vi "Handle incomming messages.vi"(11 "module loopdata":T1) -> (0 "error out":errorcluster, 3 "OK":bool)   [LabVIEW 2019, in "Communication Interface.lvlib"]
uses:
  Communication Interface.lvlib
  module data.ctl
  Intertarget communication/CR_master_class/CR_master.lvclass
  Intertarget communication/CR slave_class/CR slave.lvclass
  SubVIs/Shared/CMD Read RX.ctl
  SubVIs/Shared/CMD Read RX index.ctl
  93a0a4a7-173a-43f5-bf28-7be2535433ae.vi
  48c2df5e-f12f-4e31-93d9-71ac4fdf9692.vi
  93a0a4a7-173a-43f5-bf28-7be2535433ae.vi/fab4b5b6-9762-4187-bffd-0adbcd2d5190.vi
  93a0a4a7-173a-43f5-bf28-7be2535433ae.vi/eb0db0a0-6387-48cc-9517-445619e830de.vi
  48c2df5e-f12f-4e31-93d9-71ac4fdf9692.vi/0a35ed28-1569-4b97-93b5-a089aa938873.vi
  48c2df5e-f12f-4e31-93d9-71ac4fdf9692.vi/d25f57df-6ce4-4576-a055-01dd08f6b6ca.vi
  <vilib>/Utility/High Resolution Relative Seconds.vi
  <vilib>/Utility/error.llb/Error Cluster From Error Code.vi
  SubVIs/Shared/System GV.vi
  <vilib>/addons/_JKI.lib/Serialization/JSON/Library/Unflatten From JSON String.vi
  <vilib>/ErrorRing/Error Ring.xnode
  SubVIs/IQBurst_memo_class/IQBurst_memo.lvclass
  Intertarget communication/CommandResponse communication.lvlib
  SubVIs/Shared/Shared.lvlib
  Data Managment/DataManagment.lvlib
  <vilib>/addons/_JKI.lib/Serialization/JSON/JKI JSON Serialization.lvlib
  Log/Log.lvlib
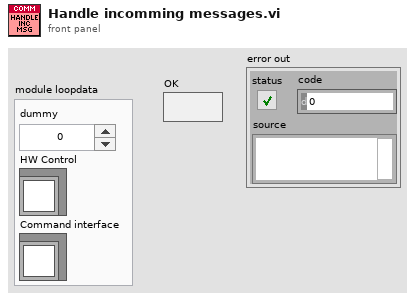
[diagram p1: front panel]
types:
  T1 = typedef "Communication Interface.lvlib/module data.ctl" = cluster{"dummy":dbl, "HW Control":refnum<class "CR_master.lvclass">, "Command interface":refnum<class "CR slave.lvclass">}
  T2 = typedef "Shared.lvlib/CMD Read RX.ctl" = cluster{"burst name":string}
  T3 = typedef "Shared.lvlib/CMD Read RX index.ctl" = cluster{"burst index":i32}
  T4 = typedef "Communication Interface.lvlib/message destination.ctl" = enum16{"unknown", "HW", "Data", "GUI", "Log", "Close"}
  T5 = cluster{"Boolean Round":bool, "code":i32, "source":string}
  T6 = typedef "DataManagment.lvlib/DM group info.ctl" = cluster{"group name":string, "burst names":string[], "burst sizes":dbl[], "Memory":dbl}
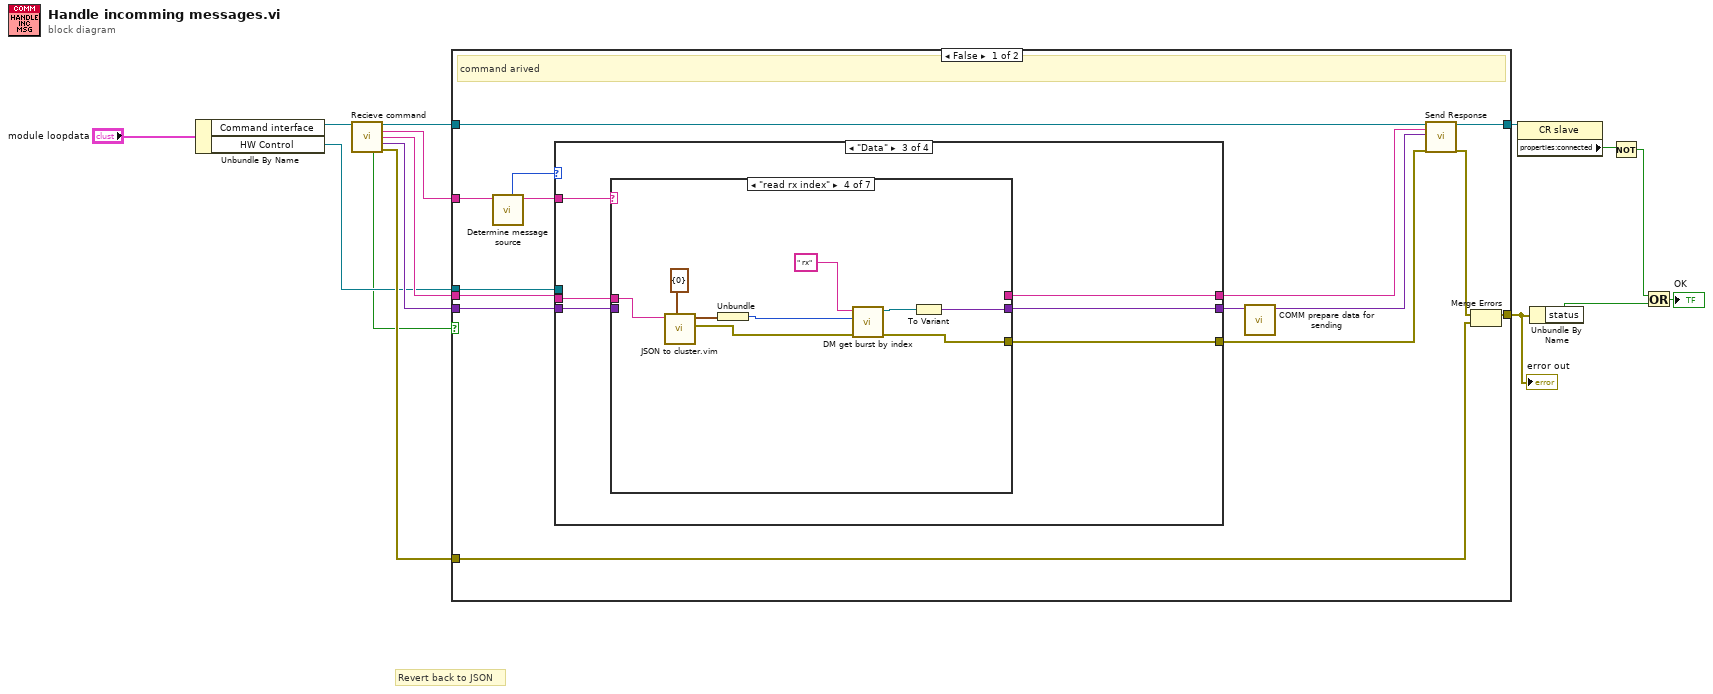
[diagram p0: block diagram]
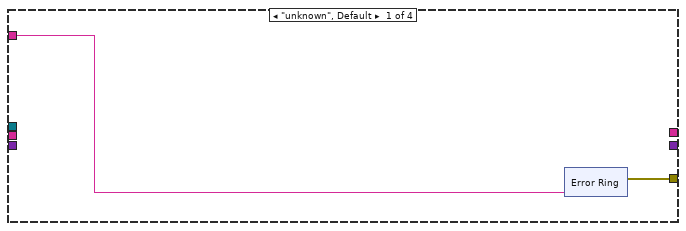
[diagram p2: hidden frame]
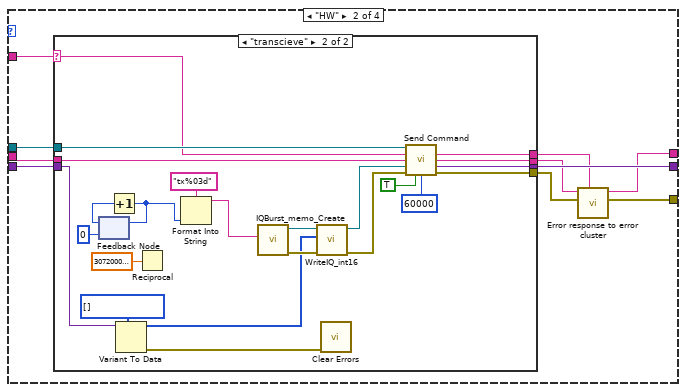
[diagram p3: hidden frame]
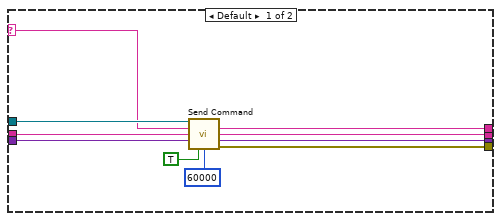
[diagram p4: hidden frame]
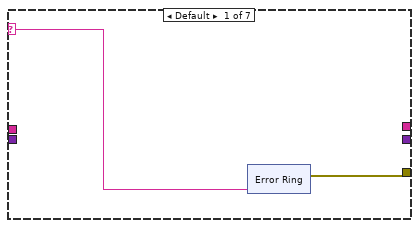
[diagram p5: hidden frame]
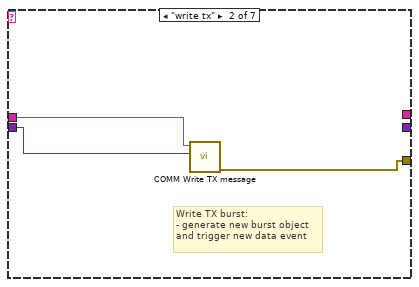
[diagram p6: hidden frame]
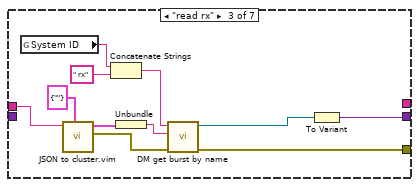
[diagram p7: hidden frame]
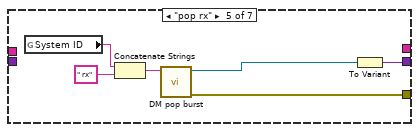
[diagram p8: hidden frame]
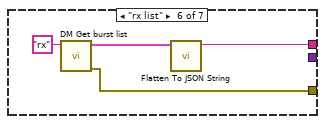
[diagram p9: hidden frame]
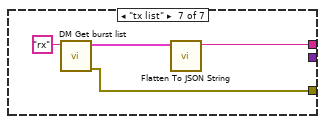
[diagram p10: hidden frame]
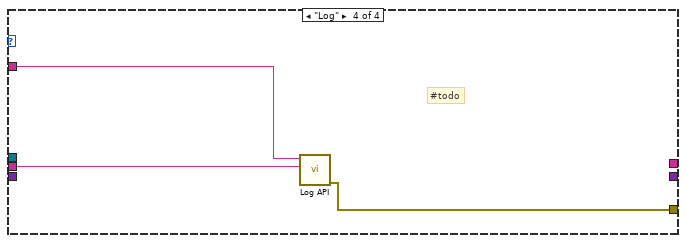
[diagram p11: hidden frame]
diagram:
  # "Revert back to JSON"
  n1 = Unbundle By Name("module loopdata") -> ("Command interface"=w2:refnum<class "CR slave.lvclass">, "HW Control"=w4:refnum<class "CR_master.lvclass">)
  n2 = call-dynamic "Recieve command.vi"("reference in"=w2) -> ("reference out"=w8:refnum<class "CR slave.lvclass">, "message"=w5:string, "parameters"=w6:string, "data"=w7:variant, "timed out?"=w3:bool, "error out"=w9:errorcluster)  [unwired: 9 in]
  n3 = case shown="False" w3 {
    tunnel: w4 -> [w30 _]
    tunnel: w5 -> [w23 _]
    tunnel: w6 -> [w29 _]
    tunnel: w7 -> [w28 _]
    tunnel: w8 -> [w27 w138]
    tunnel: w9 -> [w18 w139]
    tunnel: [w19 w139] -> w10
    tunnel: [w26 w138] -> w11
    frame False {
      # "command arived"
      n4 = call "Determine message source.vi"("message in"=w23) -> ("message out"=w22:string, "msg destination"=w21:T4)  [unwired: 9 in]
      n5 = case shown="\"Data\"" w21 {
        tunnel: w30 -> [_ w49 _ _]
        tunnel: w29 -> [_ w48 w86 w136]
        tunnel: w28 -> [_ w47 w87 _]
        tunnel: [_ w46 w84 _] -> w17
        tunnel: [_ w44 w83 _] -> w25
        tunnel: [w32 w43 w85 w135] -> w24
        tunnel: w22 -> [w31 w40 w88 w137]
        frame "unknown", Default {
          n6 = xnode "Error Ring"("parameter 0"=w31) -> ("error out"=w32:errorcluster)
        }
        frame "HW" {
          n7 = case shown="\"transcieve\"" w40 {
            selector: w40 -> [w50 w74]
            tunnel: w49 -> [w59 w82]
            tunnel: w48 -> [w58 w81]
            tunnel: w47 -> [w57 w66]
            tunnel: [w56 w80] -> w46
            tunnel: [w53 w77] -> w45
            tunnel: [w52 w76] -> w42
            tunnel: [w51 w75] -> w41
            frame Default {
              n8 = call-dynamic "Send Command.vi"("reference in"=w59, "message"=w50, "parameters"=w58, "data"=w57, "response?"=TRUE, "timeout"=60000) -> ("status"=w52:string, "reponse"=w53:string, "data"=w56:variant, "error out"=w51:errorcluster)  [unwired: 5 in, 1 out]
            }
            frame "transcieve" {
              n9 = feedback #1(0) -> (w65:i32)
              n10 = Increment(x=w65) -> (x+1=w63:i32)
              n11 = feedback-in #1(w63) -> ()
              n12 = Variant To Data(type=i16[] [], Variant=w66) -> (data=w61:i16[], error out=w73:errorcluster)  [unwired: 1 in]
              n13 = Reciprocal(x=3072000000.0 ("sample rate (Hz)")) -> ()  [unwired: 1 out]
              n14 = Format Into String(format string="tx%03d", w63) -> (resulting string=w72:string)  [unwired: 2 in, 1 out]
              n15 = call "IQBurst_memo_Create.vi"("burst name"=w72) -> ("error out"=w70:errorcluster, "reference out"=w71:refnum<class "IQBurst_memo.lvclass">)  [unwired: 9 in]
              n16 = call-dynamic "WriteIQ_int16.vi"("error in (no error)"=w70, "data"=w61, "reference in"=w71) -> ("error out"=w60:errorcluster, "reference out"=w62:refnum<class "IQBurst_memo.lvclass">)  [unwired: 7 in]
              n17 = call <vilib>:"Clear Errors.vi"("error in (no error)"=w73) -> ()  [unwired: 5 in, 2 out]
              n18 = call-dynamic "Send Command.vi"("reference in"=w82, "message"=w74, "parameters"=w81, "data"=w62, "error in (no error)"=w60, "response?"=TRUE, "timeout"=60000) -> ("status"=w76:string, "reponse"=w77:string, "data"=w80:variant, "error out"=w75:errorcluster)  [unwired: 4 in, 1 out]
            }
          }
          n19 = call "Error response to error cluster.vi"("Status"=w42, "error in (no error)"=w41, "Response in"=w45) -> ("error out"=w43:errorcluster, "Response out"=w44:string)  [unwired: 7 in]
        }
        frame "Data" {
          n20 = case shown="\"read rx index\"" w88 {
            selector: w88 -> [w90 _ _ _ _ _ _]
            tunnel: w87 -> [_ w100 _ _ _ _ _]
            tunnel: w86 -> [_ w99 w103 w116 _ _ _]
            tunnel: [w89 w98 w101 w114 w121 w128 w132] -> w85
            tunnel: [_ _ w109 w120 w124 _ _] -> w84
            tunnel: [_ _ _ _ _ w129 w133] -> w83
            frame Default {
              n21 = xnode "Error Ring"("parameter 0"=w90) -> ("error out"=w89:errorcluster)
            }
            frame "write tx" {
              # "Write TX burst:\n- generate new burst object\nand trigger new data event"
              n22 = call "COMM Write TX message.vi"("data"=w100, "parameters"=w99) -> ("error out"=w98:T5)  [unwired: 9 in]
            }
            frame "read rx" {
              n23 = global read "System GV.vi" "System ID"() -> (w111:string)
              n24 = call "JSON to cluster.vim"("data"=T2 {"burst name"=""} ("read rx command"), "JSON in"=w103) -> ("error out"=w104:errorcluster, "data"=w107:T2)  [unwired: 7 in, 1 out]
              n25 = Concatenate Strings(w111, " rx" ("group")) -> (w108:string)
              n26 = Unbundle(w107) -> ("burst name"=w105:string)
              n27 = call "DM get burst by name.vi"("error in (no error)"=w104, "Burst name"=w105, "group"=w108) -> ("error out"=w101:errorcluster, "TX burst"=w102:refnum<class "mmWave data.lvclass">)  [unwired: 7 in]
              n28 = To Variant(anything=w102) -> (Variant=w109:variant)
            }
            frame "read rx index" {
              n29 = call "JSON to cluster.vim"("data"=T3 {"burst index"=0} ("read rx command"), "JSON in"=w116) -> ("error out"=w117:errorcluster, "data"=w119:T3)  [unwired: 7 in, 1 out]
              n30 = Unbundle(w119) -> ("burst index"=w118:i32)
              n31 = call "DM get burst by index.vi"("error in (no error)"=w117, "Burst name"=w118, "group"=" rx") -> ("error out"=w114:errorcluster, "TX burst"=w115:refnum<class "mmWave data.lvclass">)  [unwired: 7 in]
              n32 = To Variant(anything=w115) -> (Variant=w120:variant)
            }
            frame "pop rx" {
              n33 = global read "System GV.vi" "System ID"() -> (w126:string)
              n34 = Concatenate Strings(w126, " rx" ("group")) -> (w123:string)
              n35 = call "DM pop burst.vi"("group"=w123) -> ("error out"=w121:errorcluster, "burst"=w122:refnum<class "mmWave data.lvclass">)  [unwired: 9 in]
              n36 = To Variant(anything=w122) -> (Variant=w124:variant)
            }
            frame "rx list" {
              n37 = call "DM Get burst list.vi"("burst group"="rx") -> ("error out"=w128:errorcluster, "burst info"=w130:T6)  [unwired: 9 in]
              n38 = call <vilib>:"Flatten To JSON String.vi"("Variant"=w130) -> ("JSON String"=w129:string)  [unwired: 9 in, 1 out]
            }
            frame "tx list" {
              n39 = call "DM Get burst list.vi"("burst group"="rx") -> ("error out"=w132:errorcluster, "burst info"=w134:T6)  [unwired: 9 in]
              n40 = call <vilib>:"Flatten To JSON String.vi"("Variant"=w134) -> ("JSON String"=w133:string)  [unwired: 9 in, 1 out]
            }
          }
        }
        frame "Log" {
          # "#todo"
          n41 = call "Log API.vi"("data"=w136, "message"=w137) -> ("error out"=w135:T5)  [unwired: 9 in]
        }
      }
      n42 = call "COMM prepare data for sending.vi"("data in"=w17) -> ("data out"=w16:variant)  [unwired: 10 in]
      n43 = call-dynamic "Send Response.vi"("reference in"=w27, "response"=w25, "data"=w16, "error in (no error)"=w24) -> ("reference out"=w26:refnum<class "CR slave.lvclass">, "error out"=w20:errorcluster)  [unwired: 14 in]
      n44 = Merge Errors(w20, w18) -> (w19:errorcluster)
    }
    frame True {
      # "timeout"
    }
  }
  "error out" <- w10
  n45 = property class="CR slave"(reference=w11) -> ("properties:connected"=w12:bool)  [unwired: 1 in, 2 out]
  n46 = Unbundle By Name(w10) -> ("status"=w13:bool)
  n47 = Not(x=w12) -> (.not. x?=w14:bool)
  n48 = Or(x=w14, y=w13) -> (x .or. y?=→"OK":bool)
